vi "KE622x -- Set List Sweep Params.vi"(0 "Resource In":refnum<visa-resource-name>, 1 "Check For SCPI Errors? (T)":bool=TRUE, 7 "List Sweep Params In":T1 {"List Sweep Steps"."Current Level (A)" min=-0.105 max=0.105 format="%.4p"; "List Sweep Steps"."Source Delay (s)" min=0.001 max=1000.0 step=0.001 format="%.3f"; "List Sweep Steps"."Voltage Limit (V)" min=0.1 max=105.0 step=0.01 format="%.2p"}, 11 "error in (no error)":errorcluster, 12 "Read Back Set Values? (T)":bool=TRUE) -> (4 "Resource Out (dupl)":refnum<visa-resource-name>, 8 "List Sweep Params Out":T1 {"List Sweep Steps"."Current Level (A)" min=-0.105 max=0.105 format="%.4p"; "List Sweep Steps"."Source Delay (s)" min=0.001 max=1000.0 step=0.001 format="%.3f"; "List Sweep Steps"."Voltage Limit (V)" min=0.1 max=105.0 step=0.01 format="%.2p"}, 15 "error out":errorcluster)   [LabVIEW 2019, in "Keithley 622x.lvlib"]
doc: "Sets up the individual points in a list current sweep and also whether or not the list current sweep will abort on a compliance (voltage limit) condition."
uses:
  Keithley 622x.lvlib
  Typedefs/KE622x -- List Sweep Params.ctl
  Typedefs/KE622x -- List Sweep Steps.ctl
  Typedefs/KE622x -- List Sweep Step.ctl
  Typedefs/KE622x -- Current Level.ctl
  Typedefs/KE622x -- Source Delay.ctl
  Typedefs/KE622x -- Voltage Limit.ctl
  Typedefs/KE622x -- Current Range.ctl
  Typedefs/KE622x -- Current Ranges.ctl
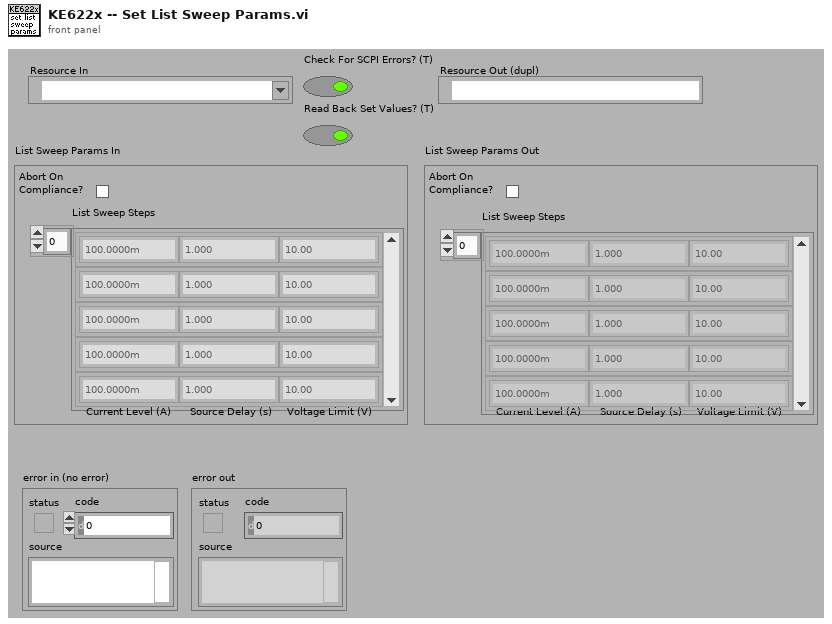
[diagram p1: front panel]
types:
  T1 = typedef "Keithley 622x.lvlib/KE622x -- List Sweep Params.ctl" = cluster{"Abort On\nCompliance?":bool, "List Sweep Steps":T2}
  T2 = typedef "Keithley 622x.lvlib/KE622x -- List Sweep Steps.ctl" = T3[]
  T3 = typedef "Keithley 622x.lvlib/KE622x -- List Sweep Step.ctl" = cluster{"Current Level (A)":T4, "Source Delay (s)":T5, "Voltage Limit (V)":T6}
  T4 = typedef "Keithley 622x.lvlib/KE622x -- Current Level.ctl" = dbl
  T5 = typedef "Keithley 622x.lvlib/KE622x -- Source Delay.ctl" = dbl
  T6 = typedef "Keithley 622x.lvlib/KE622x -- Voltage Limit.ctl" = dbl
  T7 = typedef "Keithley 622x.lvlib/KE622x -- Current Range.ctl" = cluster{"Auto Range?":bool, "Man / Selected\nRange":T8}
  T8 = typedef "Keithley 622x.lvlib/KE622x -- Current Ranges.ctl" = enum16{"2nA", "20nA", "200nA", "2uA", "20uA", "200uA", "2mA", "20mA", "100mA"}
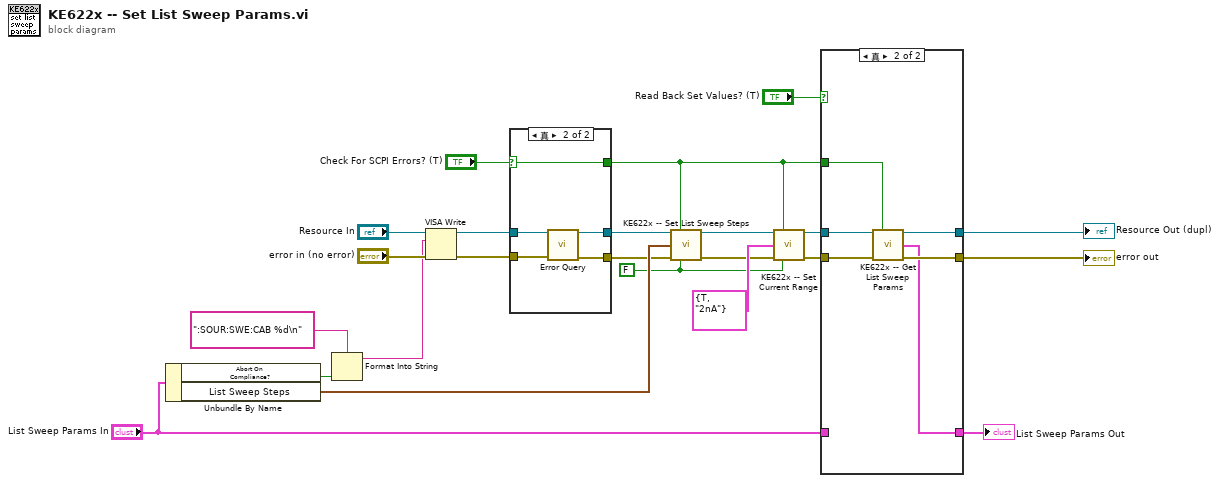
[diagram p0: block diagram]
diagram:
  w2 = FALSE ("Read Back Set Values? (T)")
  n1 = Unbundle By Name("List Sweep Params In") -> ("Abort On\nCompliance?"=w17:bool, "List Sweep Steps"=w12:T2)
  n2 = Format Into String(format string=":SOUR:SWE:CAB %d\n", w17) -> (resulting string=w16:string)  [unwired: 2 in, 1 out]
  n3 = VISA Write(VISA resource name="Resource In", write buffer=w16, error in (no error)="error in (no error)") -> (VISA resource name out=w15:refnum<visa-resource-name>, error out=w14:errorcluster)  [unwired: 1 out]
  n4 = case shown="真" "Check For SCPI Errors? (T)" {
    selector: "Check For SCPI Errors? (T)" -> [w24 w27]
    tunnel: w15 -> [w26 w31]
    tunnel: w14 -> [w25 w30]
    tunnel: [w25 w29] -> w11
    tunnel: [w26 w28] -> w13
    tunnel: [w24 w27] -> w1
    frame False {
    }
    frame True {
      n5 = call "Error Query.vi"("VISA Resource In"=w31, "error in (no error)"=w30) -> ("VISA Resource Out (dupl)"=w28:refnum<visa-resource-name>, "error out"=w29:errorcluster)  [unwired: 10 in, 2 out]
    }
  }
  n6 = call "KE622x -- Set List Sweep Steps.vi"("Resource In"=w13, "Check For SCPI Errors? (T)"=w1, "List Sweep Steps In"=w12, "error in (no error)"=w11, "Read Back Set Values? (T)"=w2) -> ("Resource Out (dupl)"=w4:refnum<visa-resource-name>, "error out"=w3:errorcluster)  [unwired: 8 in, 1 out]
  n7 = call "KE622x -- Set Current Range.vi"("Resource In"=w4, "Check For SCPI Errors? (T)"=w1, "Current Range In"=T7 {"Auto Range?"=TRUE, "Man / Selected\nRange"=enum."2nA"}, "error in (no error)"=w3, "Read Back Set Values? (T)"=w2) -> ("Resource Out (dupl)"=w7:refnum<visa-resource-name>, "error out"=w6:errorcluster)  [unwired: 8 in, 1 out]
  n8 = case shown="真" "Read Back Set Values? (T)" {
    tunnel: [w32 w40] -> w20
    tunnel: [w33 w39] -> w19
    tunnel: w1 -> [_ w38]
    tunnel: w6 -> [w32 w37]
    tunnel: w7 -> [w33 w36]
    tunnel: "List Sweep Params In" -> [w34 _]
    tunnel: [w34 w35] -> w8
    frame False {
    }
    frame True {
      n9 = call "KE622x -- Get List Sweep Params.vi"("Resource In"=w36, "Check For SCPI Errors? (T)"=w38, "error in (no error)"=w37) -> ("Resource Out (dupl)"=w39:refnum<visa-resource-name>, "List Sweep Params"=w35:T1, "error out"=w40:errorcluster)  [unwired: 10 in]
    }
  }
  "Resource Out (dupl)" <- w19
  "error out" <- w20
  "List Sweep Params Out" <- w8
